vi "Set Switch Heater.vi"(8 "error in (no error)":errorcluster, 10 "Switch Heater":T1, 11 "Instrument.1820 in":refnum<class "Instrument.Oxford1820.lvclass">) -> (0 "error out":errorcluster, 2 "Response":string, 3 "Instrument.1820 in":refnum<class "Instrument.Oxford1820.lvclass">)   [LabVIEW 2019, in "Instrument.Oxford1820.lvclass"]
uses:
  Instrument.Oxford1820.lvclass
  <instrlib>/Mercury iXX/Public/Libraries/Magnet/Controls/Switch Heater.ctl
  Typedefs/Instrument.Oxford1820.protectedCommands-enum.ctl
  15ad919e-1920-40bd-9cc5-2fd0b0d6eef7.vi/e016805e-e674-473a-8d3c-02e90b744913.vi
  15ad919e-1920-40bd-9cc5-2fd0b0d6eef7.vi/310e303c-2eaf-435c-bca2-df2e5a42084e.vi
  <vilib>/Utility/Data Type/Get Type Information.vi
  <vilib>/JDP Science/JSONtext/JSON text to Variant.vi
  <vilib>/JDP Science/JSONtext/LVClass Serializer/JSONtext LVClass Serializer.lvclass
  <instrlib>/Mercury iXX/Public/Libraries/Magnet.lvlib
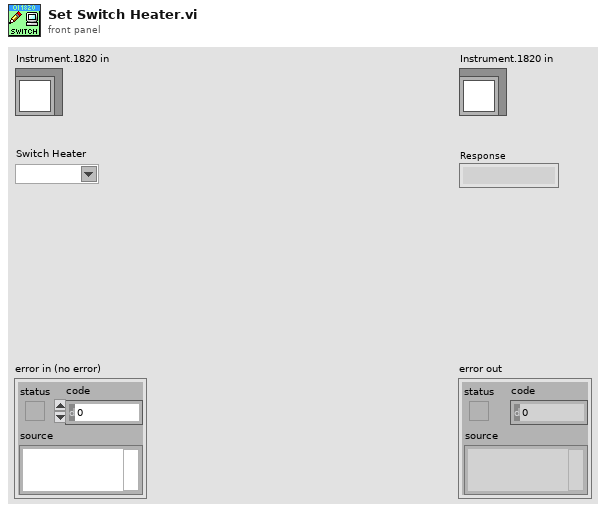
[diagram p1: front panel]
types:
  T1 = typedef "Mercury iXX.lvlib/Magnet.lvlib/Switch Heater.ctl" = string
  T2 = typedef "Instrument.Oxford1820.lvclass/Instrument.Oxford1820.protectedCommands-enum.ctl" = enum16{"Hold", "RampToSet", "RampToZero", "Clamp", "setTarget", "setSwitchHeat", "setLambda", "setFillMode", "setNeedleValve", "getStatus", "getTarget", "getSwitchHeat", "getPSUField", "setSequenceStatus"}
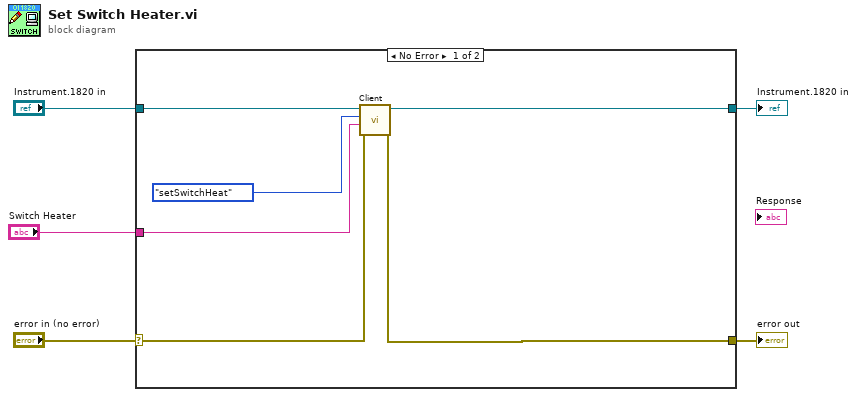
[diagram p0: block diagram]
diagram:
  n1 = case shown="No Error" "error in (no error)" {
    selector: "error in (no error)" -> [w8 w13]
    tunnel: [w6 w13] -> w4
    tunnel: [w7 w12] -> w2
    tunnel: "Instrument.1820 in" -> [w11 w12]
    tunnel: "Switch Heater" -> [w9 _]
    frame No Error {
      n2 = call-dynamic "Client.vi"("error in (no error)"=w8, "Data in"=w9, "Command in"=Instrument.Oxford1820.protectedCommands-enum."setSwitchHeat" ("Commands"), "Instrument in"=w11) -> ("error out"=w6:errorcluster, "Instrument out"=w7:refnum<class "Instrument.Oxford1820.lvclass">)  [unwired: 4 in, 2 out]
    }
    frame Error {
    }
  }
  "error out" <- w4
  "Instrument.1820 in" <- w2
